vi "E3643A_Idd Volt_Config.vi"(6 "On/Off":bool=TRUE, 8 "error in (no error)":errorcluster, 9 "Idd Limit(mA)":dbl=0.02, 10 "Volts (V)":dbl, 11 "VISA resource name":refnum<visa-resource-name>) -> (0 "error out":errorcluster, 3 "VISA resource name out":refnum<visa-resource-name>)   [LabVIEW 2012]
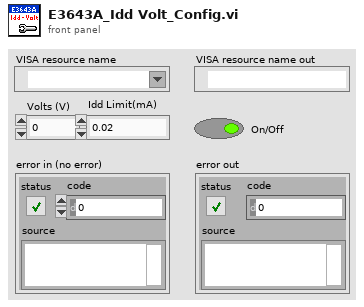
[diagram p1: front panel]
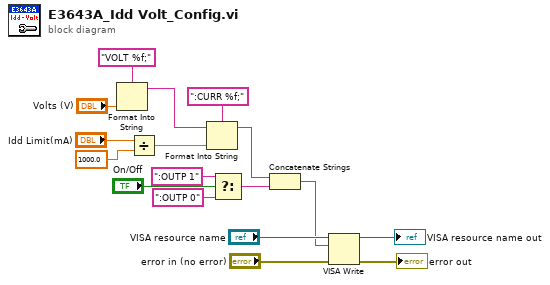
[diagram p0: block diagram]
diagram:
  n1 = Format Into String(format string="VOLT %f;", "Volts (V)") -> (resulting string=w8:string)  [unwired: 2 in, 1 out]
  n2 = Divide(x="Idd Limit(mA)", y=1000.0) -> (x/y=w1:dbl)
  n3 = Format Into String(format string=":CURR %f;", initial string=w8, w1) -> (resulting string=w5:string)  [unwired: 1 in, 1 out]
  n4 = Select(t=":OUTP 1", s="On/Off", f=":OUTP 0") -> (s? t:f=w4:string)
  n5 = Concatenate Strings(w5, w4) -> (w6:string)
  n6 = VISA Write(VISA resource name="VISA resource name", write buffer=w6, error in (no error)="error in (no error)") -> (VISA resource name out=→"VISA resource name out":refnum<visa-resource-name>, error out=→"error out":errorcluster)  [unwired: 1 out]
